vi "Case Structure.vi"() -> ()   [LabVIEW 2019]
panel:
  in  "Str Ctrl":string
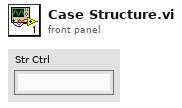
[diagram p1: front panel]
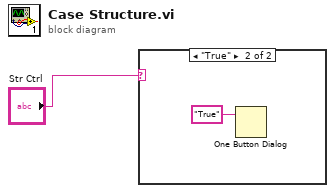
[diagram p0: block diagram]
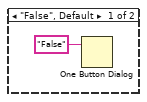
[diagram p2: hidden frame]
diagram:
  n1 = case shown="\"True\"" "Str Ctrl" {
    frame "False", Default {
      n2 = One Button Dialog(message="False") -> ()  [unwired: 1 in, 1 out]
    }
    frame "True" {
      n3 = One Button Dialog(message="True") -> ()  [unwired: 1 in, 1 out]
    }
  }
